vi "init_plotter.vi"(9 "Plot Tree":refnum<vi>, 10 "#Lines Plot":refnum<vi>, 11 "Output Files Path":refnum<vi>) -> ()   [LabVIEW 2019]
uses:
  lib/libOutputReader.so
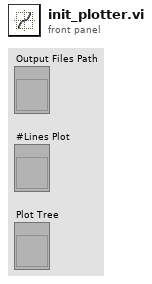
[diagram p1: front panel]
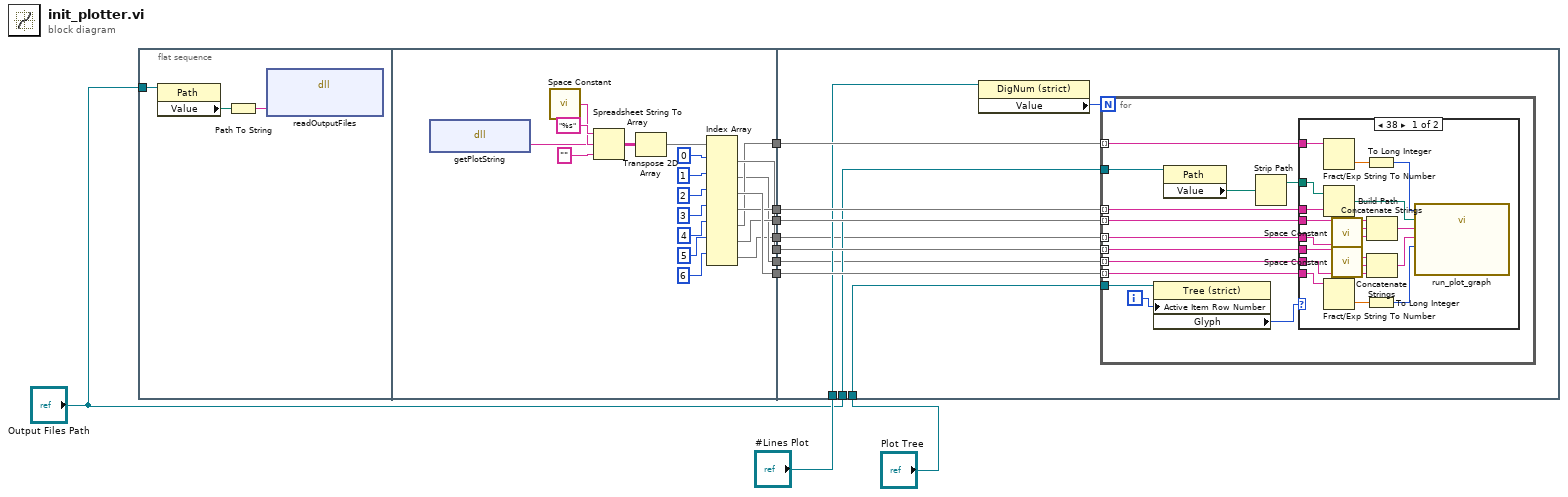
[diagram p0: block diagram]
diagram:
  n1 = flat-sequence {
    tunnel: "Output Files Path" -> [w11]
    tunnel: [w18] -> w10
    tunnel: [w17] -> w9
    tunnel: [w27] -> w8
    tunnel: [w16] -> w7
    tunnel: [w19] -> w3
    tunnel: [w15] -> w2
    tunnel: [w14] -> w1
    tunnel: w10 -> [w43]
    tunnel: w9 -> [w41]
    tunnel: w8 -> [w40]
    tunnel: w7 -> [w39]
    tunnel: "#Lines Plot" -> [w38]
    tunnel: "Output Files Path" -> [w37]
    tunnel: "Plot Tree" -> [w36]
    tunnel: w3 -> [w42]
    tunnel: w2 -> [w35]
    tunnel: w1 -> [w34]
    frame #0 {
      n2 = property class="Path"(reference=w11) -> ("Value"=w12:path)  [unwired: 1 in, 2 out]
      n3 = Path To String(path=w12) -> (string=w13:string)
      n4 = dll-call lib="home/paul/Schreibtisch/Biogas_plant_setup/lib/libOutputReader.so" fn="readOutputFiles"("pathToOutputFiles"=w13) -> ()  [unwired: 5 in, 2 out]
    }
    frame #1 {
      n5 = dll-call lib="home/paul/Schreibtisch/Biogas_plant_setup/lib/libOutputReader.so" fn="getPlotString"() -> ("plotValuesString"=w28:string)  [unwired: 3 in, 2 out]
      n6 = call <vilib>:"Space Constant.vi"() -> ("String"=w30:string)
      n7 = Spreadsheet String To Array(delimiter (Tab)=w30, format string="%s", spreadsheet string=w28, array type (2D Dbl)="") -> (array=w31:string[][])
      n8 = Transpose 2D Array(2D array=w31) -> (transposed array=w26:string[][])
      n9 = Index Array(array=w26, index (row) #1=0 ("index (row)"), index (row) #2=1 ("index (row)"), index (row) #3=2 ("index (row)"), index (row) #4=3 ("index (row)"), index (row) #5=4 ("index (row)"), index (row) #6=5 ("index (row)"), index (row) #7=6 ("index (row)")) -> (element #1=w27:string[], element #2=w15:string[], element #3=w19:string[], element #4=w18:string[], element #5=w17:string[], element #6=w16:string[], element #7=w14:string[])  [unwired: 7 in]
    }
    frame #2 {
      n10 = property class="DigNum (strict)"(reference=w38) -> ("Value"=w44:i32)  [unwired: 1 in, 2 out]
      n11 = for {
        N: w44 -> [_]
        tunnel: w43 -> [w56] mode=indexing
        tunnel: w42 -> [w52] mode=indexing
        tunnel: w41 -> [w51] mode=indexing
        tunnel: w40 -> [w50] mode=indexing
        tunnel: w39 -> [w49] mode=indexing
        tunnel: w36 -> [w48]
        tunnel: w37 -> [w47]
        tunnel: w35 -> [w46] mode=indexing
        tunnel: w34 -> [w45] mode=indexing
        i -> [w55]
        n12 = property on="Property Node" class="Tree (strict)"(reference=w48, "Active Item Row Number"=w55) -> ("Glyph"=w57:i32)  [unwired: 1 in, 2 out]
        n13 = property class="Path"(reference=w47) -> ("Value"=w54:path)  [unwired: 1 in, 2 out]
        n14 = Strip Path(path=w54) -> (stripped path=w53:path)  [unwired: 1 out]
        n15 = case shown="38" w57 {
          tunnel: w56 -> [w62 _]
          tunnel: w53 -> [w74 _]
          tunnel: w52 -> [w64 _]
          tunnel: w51 -> [w63 _]
          tunnel: w50 -> [w59 _]
          tunnel: w49 -> [w61 _]
          tunnel: w46 -> [w58 _]
          tunnel: w45 -> [w60 _]
          frame 38 {
            n16 = Fract/Exp String To Number(string=w63) -> (number=w72:dbl)  [unwired: 3 in, 1 out]
            n17 = Build Path(base path=w74, name or relative path=w62) -> (appended path=w73:path)
            n18 = Fract/Exp String To Number(string=w64) -> (number=w70:dbl)  [unwired: 3 in, 1 out]
            n19 = call <vilib>:"Space Constant.vi"() -> ("String"=w66:string)
            n20 = call <vilib>:"Space Constant.vi"() -> ("String"=w68:string)
            n21 = To Long Integer(number=w72) -> (32bit integer=w71:i32)
            n22 = To Long Integer(number=w70) -> (32bit integer=w69:i32)
            n23 = Concatenate Strings(w61, w66, w60) -> (w65:string)
            n24 = Concatenate Strings(w59, w68, w58) -> (w67:string)
            n25 = call "run_plot_graph.vi"("xValues"=w71, "yValues"=w69, "File Path"=w73, "xName"=w65, "yName"=w67) -> ()  [unwired: 6 in]
          }
          frame 15, 37, Default {
          }
        }
      }
    }
  }
